vi "Assignment1_3.vi"() -> ()   [LabVIEW 2025]
panel:
  in  "Stop":bool
  out "B":i32
  out "A":i32
  in  "Tab Control":enum32{"Page 1", "Page 2", "Page 3", "Page 4"}(tab)
  in  "N2":i32
  in  "N1":i32
  in  "N4":i32
  in  "N3":i32
  in  "N6":i32
  in  "N5":i32
  in  "N8":i32
  in  "N7":i32
  # "Page 1:  A = N1 + N2 ; B = N1 * N2\n\nPage 2:  A = N3 / N4 ; B = N3 % N4\n\nPage 3:  A = min(N5,N6) ; B = max(N5,N6) \n\nPage 4:  A = Logical Shift (N7,N8) ; Rotate(N7, N8)"
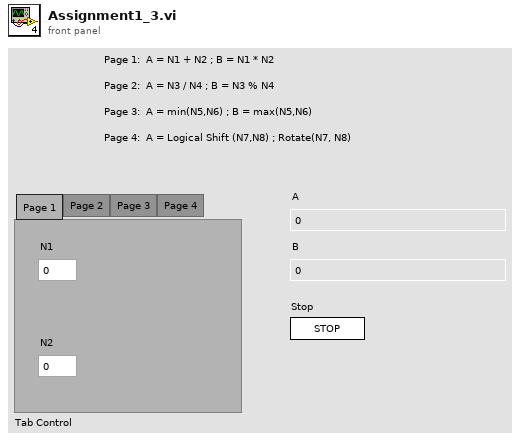
[diagram p1: front panel]
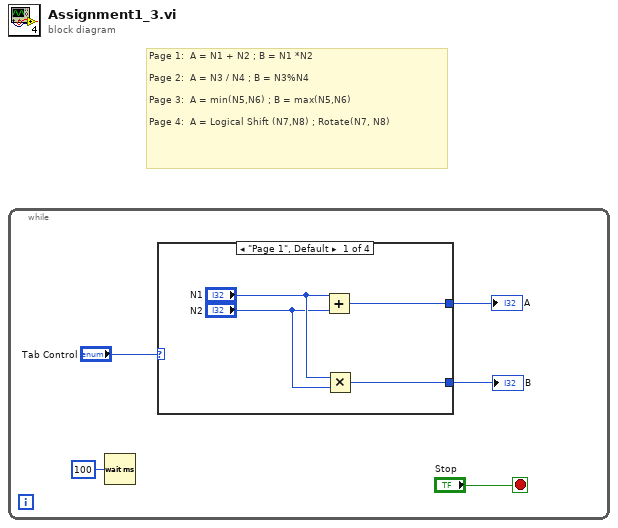
[diagram p0: block diagram]
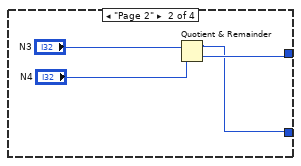
[diagram p2: hidden frame]
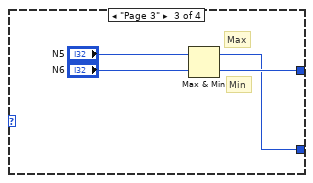
[diagram p3: hidden frame]
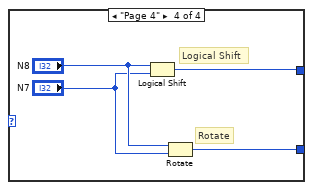
[diagram p4: hidden frame]
diagram:
  # "Page 1:  A = N1 + N2 ; B = N1 *N2\n\nPage 2:  A = N3 / N4 ; B = N3%N4\n\nPage 3:  A = min(N5,N6) ; B = max(N5,N6) \n\nPage 4:  A = Logical Shift (N7,N8) ; Rotate(N7, N8)"
  n1 = while {
    stop <- "Stop" stop-if-true
    n2 = Wait (ms)(milliseconds to wait=u32 100) -> ()  [unwired: 1 out]
    n3 = case shown="\"Page 1\", Default" "Tab Control" {
      tunnel: [w7 w11 w15 w21] -> w4
      tunnel: [w6 w10 w14 w20] -> w3
      frame "Page 1", Default {
        n4 = Add(x="N1", y="N2") -> (x+y=w7:i32)
        n5 = Multiply(x="N1", y="N2") -> (x*y=w6:i32)
      }
      frame "Page 2" {
        n6 = Quotient & Remainder(x="N3", y="N4") -> (x-y*floor(x/y)=w10:i32, floor(x/y)=w11:i32)
      }
      frame "Page 3" {
        # "Min"
        # "Max"
        n7 = Max & Min(x="N5", y="N6") -> (max(x,y)=w14:i32, min(x,y)=w15:i32)
      }
      frame "Page 4" {
        # "Rotate"
        # "Logical Shift"
        n8 = Logical Shift(y="N8", x="N7") -> (x << y=w21:i32)
        n9 = Rotate(1:"N7", 2:"N8") -> (0:w20:i32)
      }
    }
    "A" <- w4
    "B" <- w3
  }
